vi "HEWH SC4 Condition.vi"(7 "Condition#":T1, 8 "Error In":errorcluster, 9 "Saved Condition":T1, 10 "Current Cond":T1, 11 "Full Cutout?":bool) -> (0 "Error Out":errorcluster, 3 "Current Cond Out":T1)   [LabVIEW 2023]
uses:
  Type Definitions/HEWH Special Condition Check.ctl
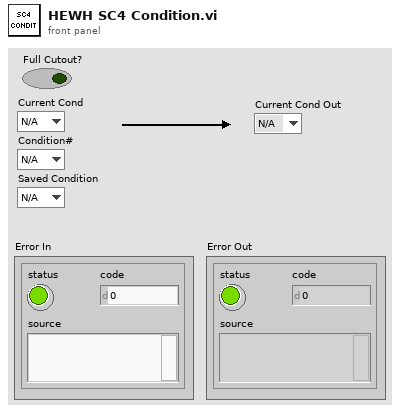
[diagram p1: front panel]
types:
  T1 = typedef "HEWH Special Condition Check.ctl" = enum16{"N/A", "C1", "C2", "Reset/Fail", "Skip Draw Sequence"}
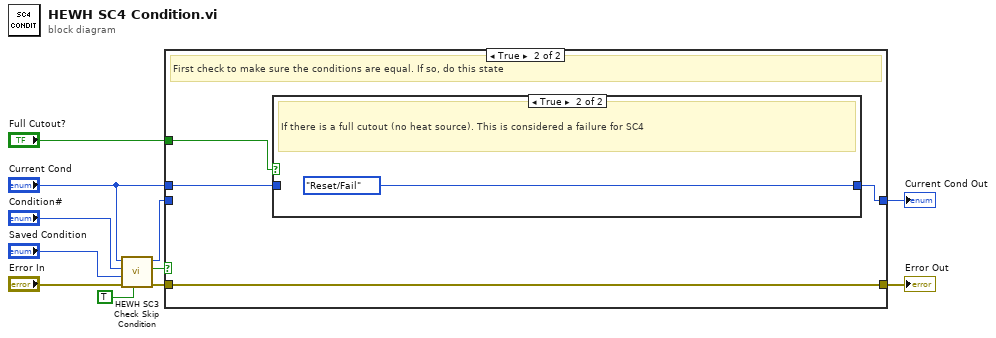
[diagram p0: block diagram]
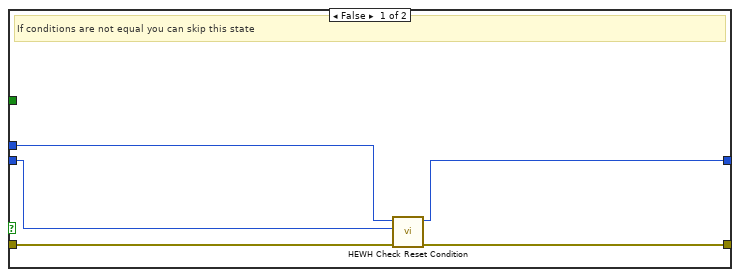
[diagram p2: hidden frame]
diagram:
  n1 = call "HEWH SC3 Check Skip Condition.vi"("Use Current Cond?"=TRUE, "Error In"="Error In", "Saved Condition"="Saved Condition", "Condition#"="Condition#", "Current Cond"="Current Cond") -> ("Error Out"=w4:errorcluster, "Conditions Equal?"=w7:bool, "SC3 Check Skip"=w6:T1)  [unwired: 4 in]
  n2 = case shown="True" w7 {
    tunnel: "Full Cutout?" -> [_ w20]
    tunnel: [w14 w19] -> w10
    tunnel: "Current Cond" -> [w16 w18]
    tunnel: w6 -> [w15 _]
    tunnel: [w12 w17] -> w3
    tunnel: w4 -> [w13 w17]
    frame False {
      # "If conditions are not equal you can skip this state"
      n3 = call "HEWH Check Reset Condition.vi"("Error In"=w13, "SC3 Check Skip"=w15, "Current Cond"=w16) -> ("Error Out"=w12:errorcluster, "Current Cond"=w14:T1)  [unwired: 6 in, 1 out]
    }
    frame True {
      # "First check to make sure the conditions are equal. If so, do this state"
      n4 = case shown="True" w20 {
        tunnel: [w21 HEWH_Special_Condition_Check."Reset/Fail" ("Special Cond Seq")] -> w19
        tunnel: w18 -> [w21 _]
        frame False {
          # "If the unit is still heating and it meets these conditions, go ahead and keep the same conditions"
        }
        frame True {
          # "If there is a full cutout (no heat source). This is considered a failure for SC4"
        }
      }
    }
  }
  "Current Cond Out" <- w10
  "Error Out" <- w3
